vi "Append Control Image to Report.vi"(0 "report in":refnum<class "NI_Standard Report.lvclass">, 1 "alignment (default)":T2, 2 "image file type (.jpg)":enum16{".jpg", ".png"}(ring), 5 "image depth":T1=2 items=["B&W", "4 bits", "8 bits", "24 bits"], 7 "ctrl reference":refnum<vi>, 9 "description":string, 11 "error in (no error)":errorcluster, 12 "MS Office parameters":T3) -> (4 "report out":refnum<class "NI_Standard Report.lvclass">, 8 "start out (Word)":i32, 10 "end out (Word)":i32, 15 "error out":errorcluster)   [LabVIEW 2017, in "NI_Standard Report.lvclass"]
doc: "Creates an image of the front panel object specified in <B>Ctrl Reference</B> and appends it to a report."
uses:
  <vilib>/Utility/NIReport.llb/Standard Report/NI_Standard Report.lvclass
  <vilib>/Utility/NIReport.llb/HTML Report Image Alignment.ctl
  <vilib>/Utility/NIReport.llb/image depth.ctl
  <vilib>/Utility/NIReport.llb/Standard Report/NI_Standard Report.lvclass/NI_Standard Report.ctl
  <vilib>/Utility/NIReport.llb/NI_ReportGenerationCore.lvlib
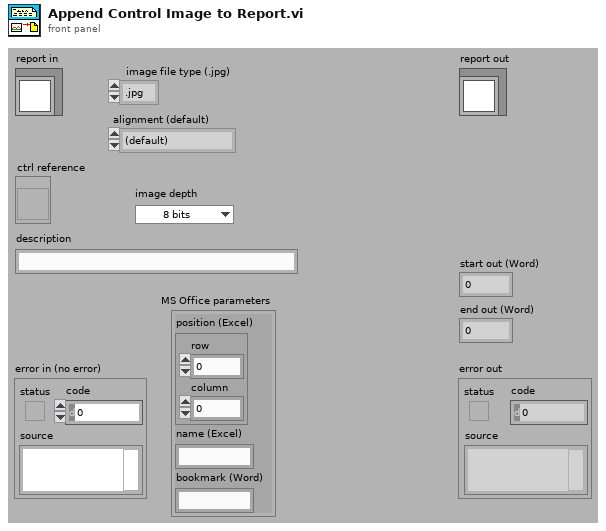
[diagram p1: front panel]
types:
  T1 = typedef "NI_ReportGenerationCore.lvlib/image depth.ctl" = u16
  T2 = typedef "NI_ReportGenerationCore.lvlib/HTML Report Image Alignment.ctl" = enum16{"(default)", "LEFT", "RIGHT", "TOP", "TEXTTOP", "MIDDLE", "ABSMIDDLE", "BASELINE", "BOTTOM", "ABSBOTTOM"}
  T3 = cluster{"position (Excel)":cluster{"row":i32, "column":i32}, "name (Excel)":string, "bookmark (Word)":string}
  T4 = typedef "imagedata.ctl" = cluster{"image type":i32, "image depth":i32, "image":u8[], "mask":u8[], "colors":u32[], "Rectangle":cluster{"left":i16, "top":i16, "right":i16, "bottom":i16}}
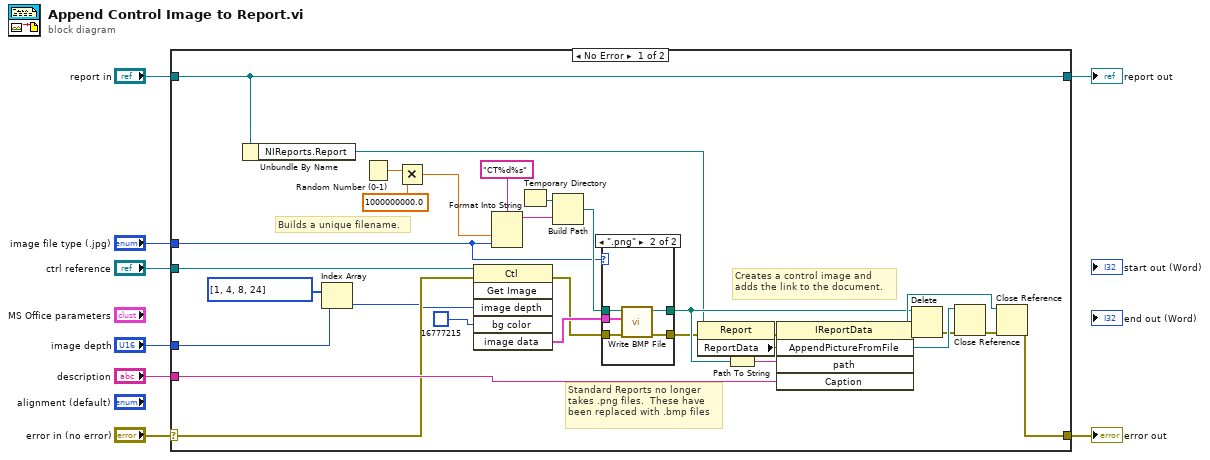
[diagram p0: block diagram]
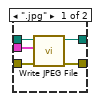
[diagram p2: hidden frame]
diagram:
  n1 = case shown="No Error" "error in (no error)" {
    selector: "error in (no error)" -> [w17 w50]
    tunnel: [w16 w50] -> w7
    tunnel: [w12 w49] -> w5
    tunnel: "report in" -> [w12 w49]
    tunnel: "ctrl reference" -> [w20 _]
    tunnel: "image file type (.jpg)" -> [w19 _]
    tunnel: "description" -> [w18 _]
    tunnel: "image depth" -> [w14 _]
    frame No Error {
      # "Standard Reports no longer\ntakes .png files.  These have\nbeen replaced with .bmp files"
      # "Builds a unique filename."
      # "Creates a control image and\nadds the link to the document."
      n2 = Unbundle By Name(w12) -> ("NIReports.Report"=w21:refnum<k7>)
      n3 = Index Array(array=i32[] [1, 4, 8, 24] ("Array Constant"), index=w14) -> (element=w13:i32)
      n4 = Random Number (0-1)() -> (number: 0 to 1=w11:dbl)
      n5 = Multiply(x=w11, y=1000000000.0) -> (x*y=w9:dbl)
      n6 = invoke class="Ctl" method="Get Image"(reference=w20, error in=w17, "image depth"=w13, "bg color"=u32 16777215) -> (error out=w32:errorcluster, "image data"=w38:T4)  [unwired: 2 in, 4 out]
      n7 = Format Into String(format string="CT%d%s" ("Format String"), w9, w19) -> (resulting string=w24:string)  [unwired: 2 in, 1 out]
      n8 = Temporary Directory() -> (w22:path)
      n9 = Build Path(base path=w22, name or relative path=w24) -> (appended path=w37:path)
      n10 = case shown="\".png\"" w19 {
        tunnel: w32 -> [w43 w46]
        tunnel: [w42 w45] -> w26
        tunnel: w37 -> [w40 w48]
        tunnel: [w41 w44] -> w29
        tunnel: w38 -> [w39 w47]
        frame ".jpg" {
          n11 = call <vilib>:"Write JPEG File.vi"("error in (no error)"=w43, "image data"=w39, "path to JPEG file"=w40) -> ("error out"=w42:errorcluster, "path"=w41:path)  [unwired: 7 out]
        }
        frame ".png" {
          n12 = call <vilib>:"Write BMP File.vi"("error in (no error)"=w46, "image data"=w47, "path to BMP file"=w48) -> ("error out"=w45:errorcluster, "path"=w44:path)  [unwired: 7 out]
        }
      }
      n13 = property class="Report"(reference=w21, error in=w26) -> (error out=w27:errorcluster, "ReportData"=w25:refnum<k7>)  [unwired: 1 out]
      n14 = Path To String(path=w29) -> (string=w28:string)
      n15 = invoke class="IReportData" method="AppendPictureFromFile"(reference=w25, error in=w27, "path"=w28, "Caption"=w18) -> (reference out=w36:refnum<k7>, error out=w30:errorcluster, "AppendPictureFromFile"=w35:refnum<k7>)  [unwired: 1 in, 2 out]
      n16 = Delete(path (use dialog)=w29, error in=w30) -> (error out=w33:errorcluster)  [unwired: 5 out]
      n17 = Close Reference(reference=w35, error in (no error)=w33) -> (error out=w34:errorcluster)
      n18 = Close Reference(reference=w36, error in (no error)=w34) -> (error out=w16:errorcluster)
    }
    frame Error {
    }
  }
  "error out" <- w7
  "report out" <- w5
